vi "Start Timer.vi"(8 "error in (no error)":errorcluster, 11 "Timer Demo App in":refnum<class "Timer Demo App.lvclass">) -> (0 "error out":errorcluster, 3 "Timer Demo App out":refnum<class "Timer Demo App.lvclass">)   [LabVIEW 2020, in "Timer Demo.lvlib" / "Timer Demo App.lvclass"]
uses:
  Timer Demo App.lvclass
  Timer Demo App.lvclass/Timer Demo App.ctl
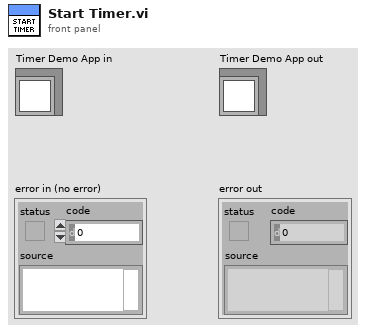
[diagram p1: front panel]
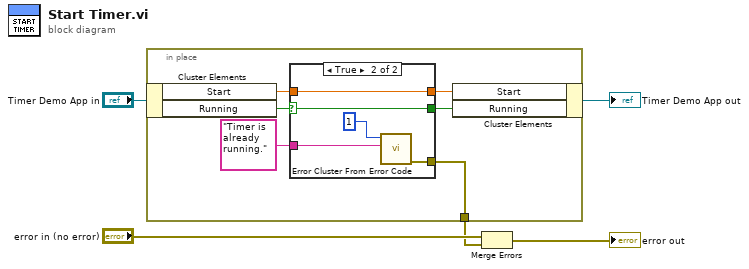
[diagram p0: block diagram]
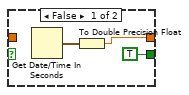
[diagram p2: hidden frame]
diagram:
  n1 = in-place {
    in-place-border: [w6] -> w1
    n2 = in-place-cluster #1("Timer Demo App in") -> ("Start"=w10:dbl, "Running"=w11:bool)
    n3 = case shown="True" w11 {
      selector: w11 -> [_ w18]
      tunnel: w10 -> [_ w19]
      tunnel: [w13 w19] -> w9
      tunnel: [TRUE w18] -> w8
      tunnel: "Timer is already running." ("error message (\"\")") -> [_ w16]
      tunnel: [_ w15] -> w6
      frame False {
        n4 = Get Date/Time In Seconds() -> (seconds since 1Jan1904=w14:timestamp)
        n5 = To Double Precision Float(number=w14) -> (double precision float=w13:dbl)
      }
      frame True {
        n6 = call <vilib>:"Error Cluster From Error Code.vi"("error message (\"\")"=w16, "error code (0)"=1) -> ("error out"=w15:errorcluster)  [unwired: 7 in]
      }
    }
    n7 = in-place-cluster #1("Start"=w9, "Running"=w8) -> (→"Timer Demo App out":refnum<class "Timer Demo App.lvclass">)
  }
  n8 = Merge Errors("error in (no error)", w1) -> (→"error out":errorcluster)
